vi "Is Connected.vi"(8 "error in (no error)":errorcluster, 11 "StringStream in":refnum<class "StringStream.lvclass">) -> (0 "error out":errorcluster, 2 "Connected":bool, 3 "StringStream out":refnum<class "StringStream.lvclass">)   [LabVIEW 2020, in "Stream.lvlib" / "StringStream.lvclass"]
uses:
  StringStream.lvclass
  StringStream.lvclass/StringStream.ctl
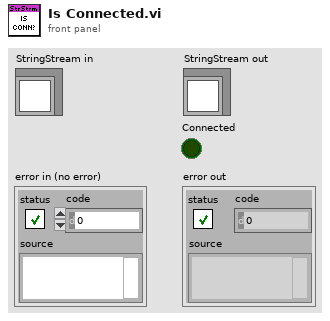
[diagram p1: front panel]
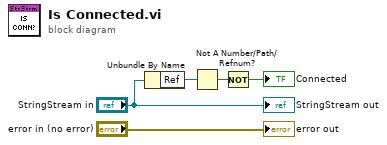
[diagram p0: block diagram]
diagram:
  n1 = Unbundle By Name("StringStream in") -> ("Ref"=w3:refnum<data-value>)
  n2 = Not A Number/Path/Refnum?(number/path/refnum=w3) -> (NaN/Path/Refnum?=w2:bool)
  n3 = Not(x=w2) -> (.not. x?=→"Connected":bool)
  "error out" <- "error in (no error)"
  "StringStream out" <- "StringStream in"
